vi "2L02-per-conv-xi-en-xic-dx.vi"(9 "xi":dbl[](array[numeric])) -> (2 "dx":dbl[](array[numeric]), 3 "xic":dbl[](array[numeric]))   [LabVIEW 2010, in "lv_02.lvlib"]
doc: "[Xi] contient les limites des classe d'une distribution MIF\nLe vi calcule le centre [Xic] et la longueur de chaque classe [dx]"
uses:
  lv_02.lvlib
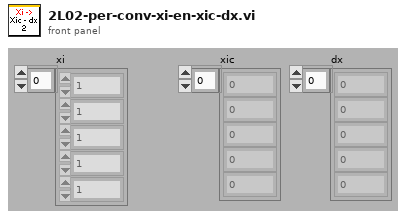
[diagram p1: front panel]
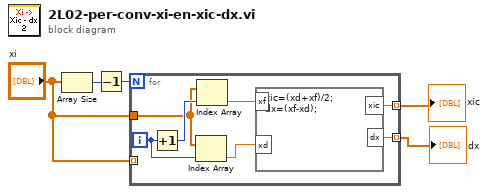
[diagram p0: block diagram]
diagram:
  n1 = Array Size(array="xi") -> (size(s)=w5:i32)
  n2 = Decrement(x=w5) -> (x-1=w4:i32)
  n3 = for {
    N: w4 -> [_]
    tunnel: "xi" -> [w11]
    tunnel: [w7] -> w3 mode=indexing
    tunnel: [w6] -> w2 mode=indexing
    tunnel: "xi" -> [_] mode=indexing
    i -> [w10]
    n4 = Increment(x=w10) -> (x+1=w12:i32)
    n5 = Index Array(array=w11, index=w10) -> (element=w8:dbl)
    n6 = Index Array(array=w11, index=w12) -> (element=w9:dbl)
    n7 = formula code="xic=(xd+xf)/2;\ndx=(xf-xd);"("xf"=w9, "xd"=w8) -> ("xic"=w7:dbl, "dx"=w6:dbl)
  }
  "xic" <- w3
  "dx" <- w2
